vi "On off text.vi"(11 "ON/OFF":bool) -> (3 "ON/OFF":string)   [LabVIEW 2019]
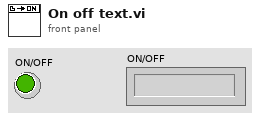
[diagram p1: front panel]
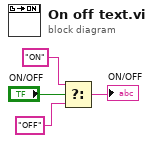
[diagram p0: block diagram]
diagram:
  n1 = Select(t="ON", s="ON/OFF", f="OFF") -> (s? t:f=→"ON/OFF":string)
